vi "Set Window Position.vi"(8 "error in (no error)":errorcluster, 10 "Current VI":refnum<vi>, 11 "Main VI":refnum<vi>) -> (0 "error out":errorcluster)   [LabVIEW 2015, in "ConfigHelper.lvlib"]
uses:
  ConfigHelper.lvlib
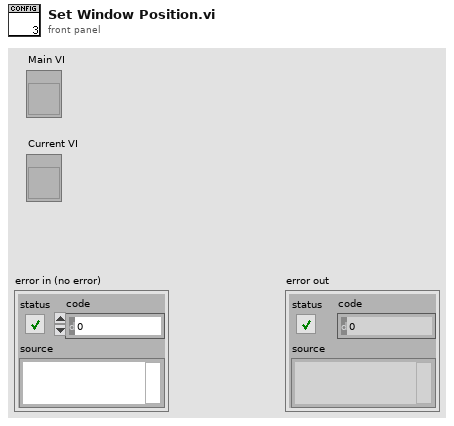
[diagram p1: front panel]
types:
  T1 = typedef "LVRectTypeDef.ctl" = cluster{"Left":i16, "Top":i16, "Right":i16, "Bottom":i16}
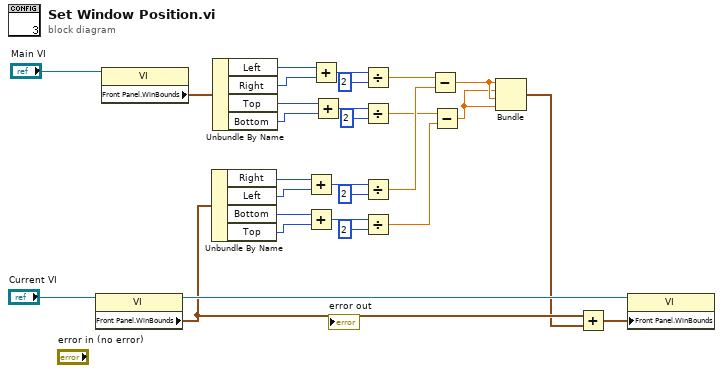
[diagram p0: block diagram]
diagram:
  n1 = property class="VI"(reference="Current VI") -> (reference out=w10:refnum<vi>, "Front Panel.WinBounds"=w3:T1)  [unwired: 1 in, 1 out]
  n2 = property class="VI"(reference="Main VI") -> ("Front Panel.WinBounds"=w28:T1)  [unwired: 1 in, 2 out]
  n3 = Unbundle By Name(w3) -> ("Right"=w18:i16, "Left"=w17:i16, "Bottom"=w16:i16, "Top"=w15:i16)
  n4 = Unbundle By Name(w28) -> ("Left"=w27:i16, "Right"=w26:i16, "Top"=w21:i16, "Bottom"=w20:i16)
  n5 = Add(x=w18, y=w17) -> (x+y=w14:i16)
  n6 = Add(x=w16, y=w15) -> (x+y=w11:i16)
  n7 = Add(x=w27, y=w26) -> (x+y=w22:i16)
  n8 = Add(x=w21, y=w20) -> (x+y=w23:i16)
  n9 = Divide(x=w22, y=i16 2) -> (x/y=w9:dbl)
  n10 = Divide(x=w23, y=i16 2) -> (x/y=w7:dbl)
  n11 = Divide(x=w14, y=i16 2) -> (x/y=w8:dbl)
  n12 = Divide(x=w11, y=i16 2) -> (x/y=w6:dbl)
  n13 = Subtract(x=w9, y=w8) -> (x-y=w5:dbl)
  n14 = Subtract(x=w7, y=w6) -> (x-y=w4:dbl)
  n15 = Bundle(w5, w4, w5, w4) -> (w1:cluster{dbl, dbl, dbl, dbl})  [unwired: 1 in]
  n16 = Add(x=w3, y=w1) -> (x+y=w2:cluster{dbl, dbl, dbl, dbl})
  n17 = property class="VI"(reference=w10, "Front Panel.WinBounds"=w2) -> ()  [unwired: 1 in, 2 out]
